vi "Receive.vi"(8 "error in (no error)":errorcluster, 9 "timeout in ms (0)":i32, 11 "Communication in":refnum<class "IP_Communication.lvclass">) -> (0 "error out":errorcluster, 1 "Timeout?":bool, 2 "Packet Received":refnum<class "Packet.lvclass">, 3 "Communication out":refnum<class "IP_Communication.lvclass">)   [LabVIEW 2020, in "Communication Classes.lvlib" / "IP_Communication.lvclass"]
uses:
  IP_Communication.lvclass
  Packet/Packet.lvclass
  IP_Communication.lvclass/IP_Communication.ctl
  <vilib>/Utility/error.llb/Error Cluster From Error Code.vi
  <vilib>/ErrorRing/Error Ring.xnode
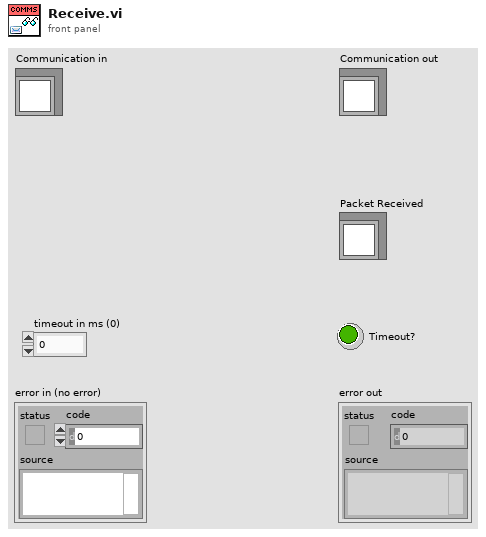
[diagram p1: front panel]
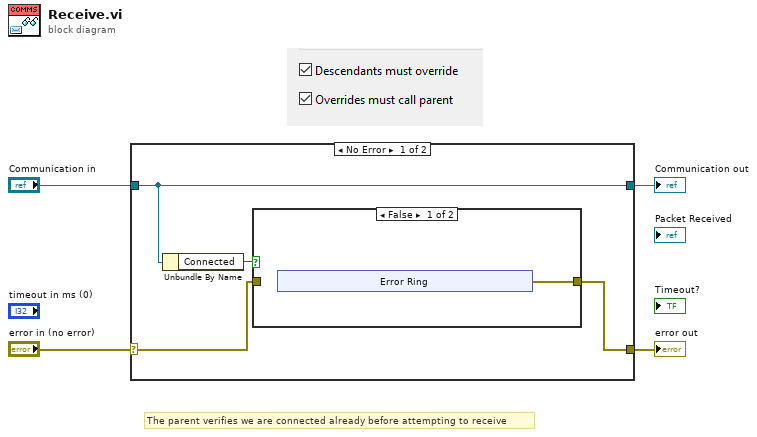
[diagram p0: block diagram]
diagram:
  # "The parent verifies we are connected already before attempting to receive"
  n1 = case shown="No Error" "error in (no error)" {
    selector: "error in (no error)" -> [w8 w17]
    tunnel: [w7 w17] -> w3
    tunnel: [w6 w16] -> w1
    tunnel: "Communication in" -> [w6 w16]
    frame No Error {
      n2 = Unbundle By Name(w6) -> ("Connected"=w5:bool)
      n3 = case shown="False" w5 {
        tunnel: w8 -> [_ w15]
        tunnel: [w9 w15] -> w7
        frame False {
          n4 = xnode "Error Ring"() -> ("error out"=w9:errorcluster)
        }
        frame True {
        }
      }
    }
    frame Error {
    }
  }
  "error out" <- w3
  "Communication out" <- w1
